vi "Scale Font.vi"(10 "scaling settings":T1={"scaling factor"={"horizontal"=1.0, "vertical"=1.0}, "scale text"=FALSE} {"scaling factor"."vertical" min=0.0; "scaling factor"."horizontal" min=0.0}, 11 "font size in":u16) -> (3 "font size out":u16)   [LabVIEW 2010, in "NI_SE_Front Panel Layout.lvlib"]
uses:
  NI_SE_Front Panel Layout.lvlib
  Scaling Factor_Options.ctl
  XY Scaling Factor.ctl
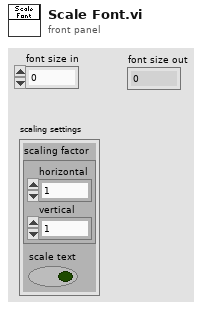
[diagram p1: front panel]
types:
  T1 = typedef "NI_SE_Front Panel Layout.lvlib/Scaling Factor_Options.ctl" = cluster{"scaling factor":T2, "scale text":bool}
  T2 = typedef "NI_SE_Front Panel Layout.lvlib/XY Scaling Factor.ctl" = cluster{"horizontal":dbl, "vertical":dbl}
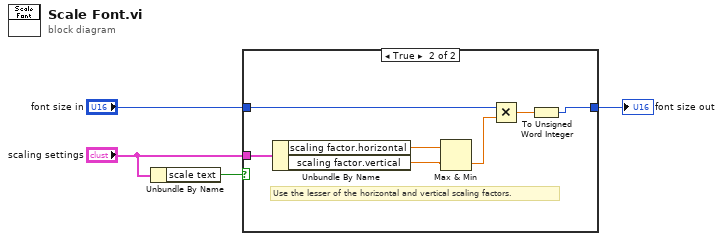
[diagram p0: block diagram]
diagram:
  n1 = Unbundle By Name("scaling settings") -> ("scale text"=w3:bool)
  n2 = case shown="True" w3 {
    tunnel: "scaling settings" -> [_ w12]
    tunnel: "font size in" -> [w5 w11]
    tunnel: [w5 w10] -> w1
    frame False {
    }
    frame True {
      # "Use the lesser of the horizontal and vertical scaling factors."
      n3 = Unbundle By Name(w12) -> ("scaling factor.horizontal"=w9:dbl, "scaling factor.vertical"=w8:dbl)
      n4 = Max & Min(x=w9, y=w8) -> (min(x,y)=w7:dbl)  [unwired: 1 out]
      n5 = Multiply(x=w11, y=w7) -> (x*y=w6:dbl)
      n6 = To Unsigned Word Integer(number=w6) -> (unsigned 16bit integer=w10:u16)
    }
  }
  "font size out" <- w1
